vi "Wait for Requesting Complete.vi"(8 "error in (no error)":errorcluster, 10 "Maximum Time (10000 ms)":i32=10000, 11 "VISA resource name":refnum<visa-resource-name>) -> (0 "error out":errorcluster, 3 "VISA resource name out":refnum<visa-resource-name>)   [LabVIEW 2014, in "Agilent U2000 Series.lvlib"]
doc: "Waits for the current requesing to finish. This VI should be called when you want to ensure a requesting(eg. calibration) has completed.\n\nNote:\nUse this VI only with other low-level VIs. The high-level VIs automatically incorporate this functionality. This VI does not check the instrument status."
uses:
  Agilent U2000 Series.lvlib
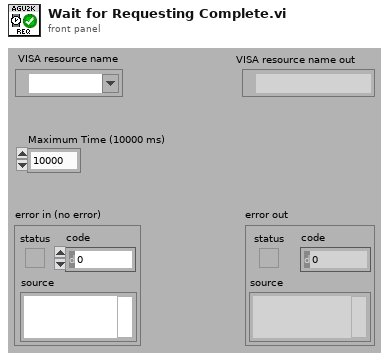
[diagram p1: front panel]
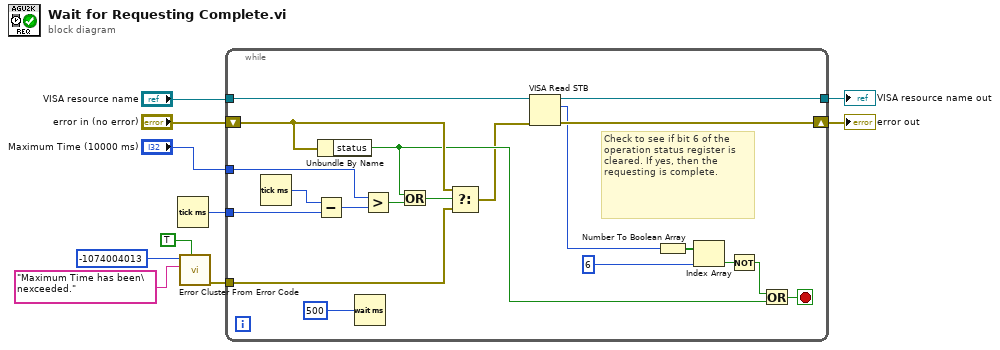
[diagram p0: block diagram]
diagram:
  n1 = Tick Count (ms)() -> (millisecond timer value=w4:u32)
  n2 = call "Error Cluster From Error Code.vi"("show call chain? (False)"=TRUE, "error message (\"\")"="Maximum Time has been\nexceeded." ("error message (\"\")"), "error code (0)"=-1074004013) -> ("error out"=w3:errorcluster)  [unwired: 1 in, 5 out]
  n3 = while {
    tunnel: [w15] -> w1
    tunnel: "VISA resource name" -> [w14]
    tunnel: "Maximum Time (10000 ms)" -> [w27]
    tunnel: w4 -> [w28]
    tunnel: w3 -> [w23]
    shift-right: [w16] -> w2
    shift-left: "error in (no error)" -> [w24]
    stop <- w22 stop-if-true
    # "Check to see if bit 6 of the operation status register is cleared. If yes, then the requesting is complete."
    n4 = Tick Count (ms)() -> (millisecond timer value=w30:u32)
    n5 = Subtract(x=w30, y=w28) -> (x-y=w29:u32)
    n6 = Unbundle By Name(w24) -> ("status"=w21:bool)
    n7 = Wait (ms)(milliseconds to wait=u32 500) -> ()  [unwired: 1 out]
    n8 = Greater?(x=w27, y=w29) -> (0:w26:bool)
    n9 = Or(x=w21, y=w26) -> (x .or. y?=w25:bool)
    n10 = Select(t=w24, s=w25, f=w23) -> (s? t:f=w17:errorcluster)
    n11 = VISA Read STB(8:w17, 11:w14) -> (0:w16:errorcluster, 2:w13:u16, 3:w15:refnum<visa-resource-name>)
    n12 = Number To Boolean Array(number=w13) -> (Boolean array=w20:bool[])
    n13 = Index Array(array=w20, index=6) -> (element=w12:bool)
    n14 = Not(x=w12) -> (.not. x?=w11:bool)
    n15 = Or(x=w11, y=w21) -> (x .or. y?=w22:bool)
  }
  "error out" <- w2
  "VISA resource name out" <- w1
